vi "foodArray.vi"(6 "element":string, 9 "Numeric":i32, 10 "element 2":string, 11 "Array in":string[][](array[string])) -> (3 "Array out":string[][](array[string]))   [LabVIEW 2015]
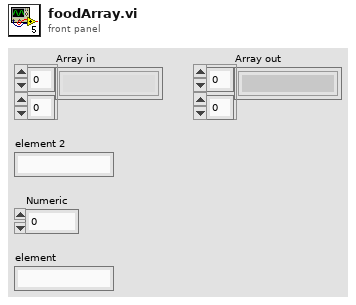
[diagram p1: front panel]
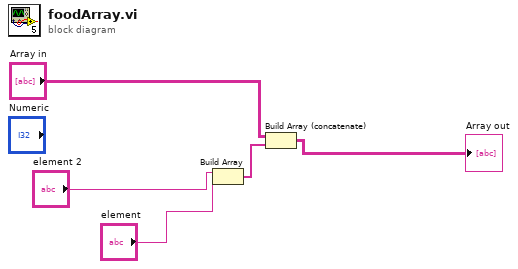
[diagram p0: block diagram]
diagram:
  n1 = Build Array("element 2", "element") -> (w4:string[])
  n2 = Build Array (concatenate)("Array in", w4) -> (→"Array out":string[][])
